vi "Fetch200HZOffsets.vi"(6 "First Segment":dbl, 7 "Number of Segments":dbl, 8 "error in (no error)":errorcluster, 10 "Source (0: Channel 1)":u16(ring) items=["Channel 1", "Channel 2", "Channel 3", "Channel 4"], 11 "VISA Resource Name in":refnum<visa-resource-name>) -> (0 "error out":errorcluster, 2 "HZ offsets":dbl[](array[numeric]), 3 "VISA Resource Name out":refnum<visa-resource-name>)   [LabVIEW 2022 SP3]
uses:
  <instrlib>/LeCroy Wave Series/LeCroy Wave Series.lvlib
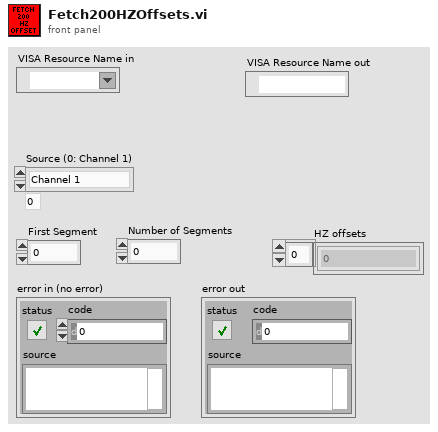
[diagram p1: front panel]
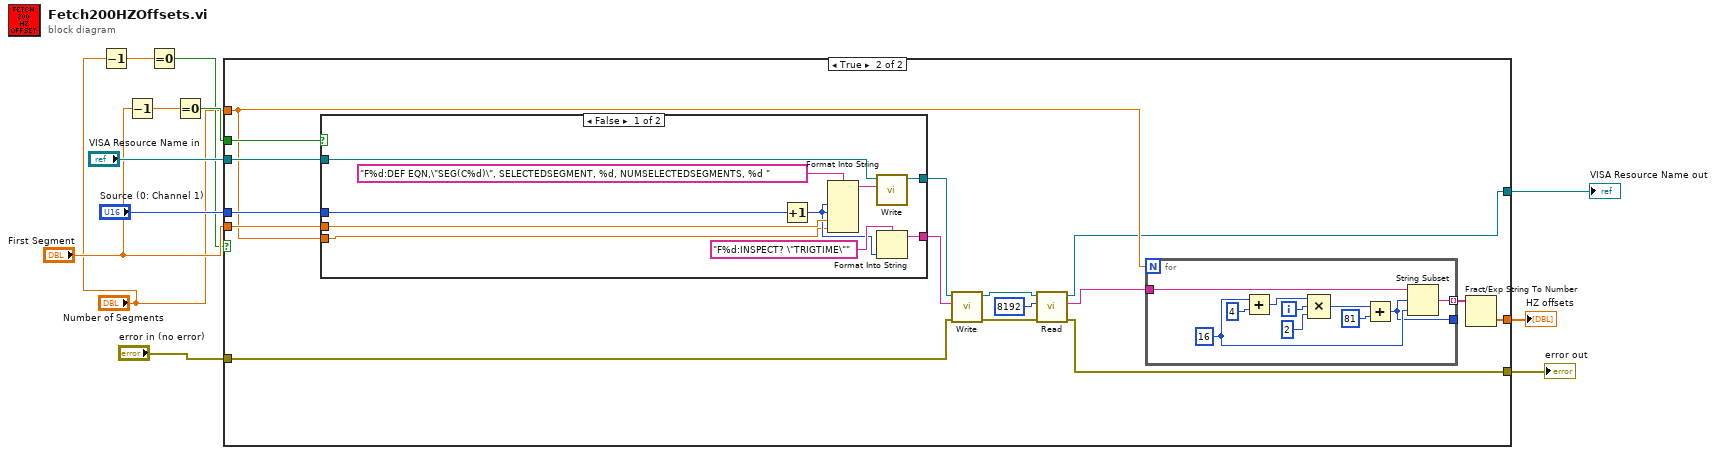
[diagram p0: block diagram]
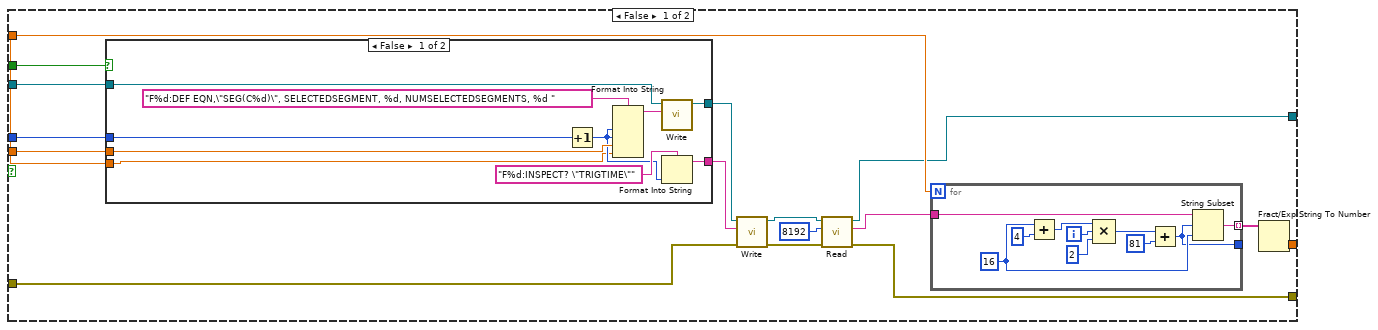
[diagram p2: hidden frame]
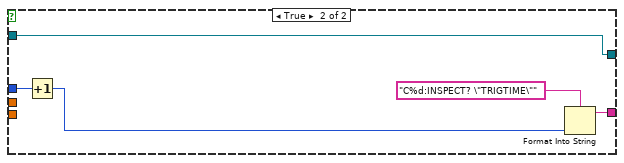
[diagram p3: hidden frame]
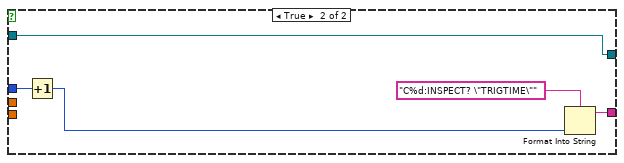
[diagram p4: hidden frame]
diagram:
  n1 = Decrement(x="Number of Segments") -> (x-1=w6:dbl)
  n2 = Decrement(x="First Segment") -> (x-1=w7:dbl)
  n3 = Equal To 0?(x=w6) -> (x = 0?=w5:bool)
  n4 = Equal To 0?(x=w7) -> (x = 0?=w9:bool)
  n5 = case shown="True" w5 {
    tunnel: "Number of Segments" -> [w28 w55]
    tunnel: "VISA Resource Name in" -> [w27 w69]
    tunnel: [w24 w66] -> w11
    tunnel: "Source (0: Channel 1)" -> [w18 w60]
    tunnel: w9 -> [w17 w59]
    tunnel: "First Segment" -> [w16 w58]
    tunnel: "error in (no error)" -> [w15 w56]
    tunnel: [w14 w57] -> w2
    tunnel: [w13 w54] -> w1
    frame False {
      n6 = case shown="False" w17 {
        tunnel: [w37 w43] -> w25
        tunnel: w27 -> [w38 w43]
        tunnel: [w35 w39] -> w26
        tunnel: w16 -> [w33 _]
        tunnel: w28 -> [w30 _]
        tunnel: w18 -> [w34 w40]
        frame False {
          n7 = Increment(x=w34) -> (x+1=w31:u16)
          n8 = Format Into String(format string="F%d:DEF EQN,\"SEG(C%d)\", SELECTEDSEGMENT, %d, NUMSELECTEDSEGMENTS, %d " ("Write Buffer"), w31, w31, w33, w30) -> (resulting string=w32:string)  [unwired: 2 in, 1 out]
          n9 = call <instrlib>:"Write.vi"("Write Buffer"=w32, "VISA resource name"=w38) -> ("VISA resource name out"=w37:refnum<visa-resource-name>)  [unwired: 7 in, 2 out]
          n10 = Format Into String(format string="F%d:INSPECT? \"TRIGTIME\"" ("Write Buffer"), w31) -> (resulting string=w35:string)  [unwired: 2 in, 1 out]
        }
        frame True {
          n11 = Increment(x=w40) -> (x+1=w42:u16)
          n12 = Format Into String(format string="C%d:INSPECT? \"TRIGTIME\"" ("Write Buffer"), w42) -> (resulting string=w39:string)  [unwired: 2 in, 1 out]
        }
      }
      n13 = call <instrlib>:"Write.vi"("error in (no error)"=w15, "Write Buffer"=w26, "VISA resource name"=w25) -> ("error out"=w19:errorcluster, "VISA resource name out"=w20:refnum<visa-resource-name>)  [unwired: 6 in, 1 out]
      n14 = call <instrlib>:"Read.vi"("error in (no error)"=w19, "Byte Count"=u32 8192, "VISA resource name"=w20) -> ("error out"=w14:errorcluster, "Read Buffer"=w22:string, "VISA resource name out"=w13:refnum<visa-resource-name>)  [unwired: 5 in, 1 out]
      n15 = for {
        N: w28 -> [_]
        tunnel: w22 -> [w52]
        tunnel: [w48] -> w23 mode=indexing
        tunnel: [w47] -> _
        i -> [w46]
        w51 = 16 ("length (rest)")
        n16 = Add(x=w51, y=4) -> (x+y=w45:i32)
        n17 = Compound Arithmetic op=MULTIPLY(w45, w46, 2 ("value")) -> (w50:i32)
        n18 = Add(x=w50, y=81 ("offset (0)")) -> (x+y=w47:i32)
        n19 = String Subset(string=w52, offset (0)=w47, length (rest)=w51) -> (substring=w48:string)
      }
      n20 = Fract/Exp String To Number(string=w23) -> (number=w24:dbl[])  [unwired: 3 in, 1 out]
    }
    frame True {
      n21 = case shown="False" w59 {
        tunnel: [w78 w84] -> w67
        tunnel: w69 -> [w79 w84]
        tunnel: [w76 w80] -> w68
        tunnel: w58 -> [w74 _]
        tunnel: w55 -> [w71 _]
        tunnel: w60 -> [w75 w81]
        frame False {
          n22 = Increment(x=w75) -> (x+1=w72:u16)
          n23 = Format Into String(format string="F%d:DEF EQN,\"SEG(C%d)\", SELECTEDSEGMENT, %d, NUMSELECTEDSEGMENTS, %d " ("Write Buffer"), w72, w72, w74, w71) -> (resulting string=w73:string)  [unwired: 2 in, 1 out]
          n24 = call <instrlib>:"Write.vi"("Write Buffer"=w73, "VISA resource name"=w79) -> ("VISA resource name out"=w78:refnum<visa-resource-name>)  [unwired: 7 in, 2 out]
          n25 = Format Into String(format string="F%d:INSPECT? \"TRIGTIME\"" ("Write Buffer"), w72) -> (resulting string=w76:string)  [unwired: 2 in, 1 out]
        }
        frame True {
          n26 = Increment(x=w81) -> (x+1=w83:u16)
          n27 = Format Into String(format string="C%d:INSPECT? \"TRIGTIME\"" ("Write Buffer"), w83) -> (resulting string=w80:string)  [unwired: 2 in, 1 out]
        }
      }
      n28 = call <instrlib>:"Write.vi"("error in (no error)"=w56, "Write Buffer"=w68, "VISA resource name"=w67) -> ("error out"=w61:errorcluster, "VISA resource name out"=w62:refnum<visa-resource-name>)  [unwired: 6 in, 1 out]
      n29 = call <instrlib>:"Read.vi"("error in (no error)"=w61, "Byte Count"=u32 8192, "VISA resource name"=w62) -> ("error out"=w57:errorcluster, "Read Buffer"=w64:string, "VISA resource name out"=w54:refnum<visa-resource-name>)  [unwired: 5 in, 1 out]
      n30 = for {
        N: w55 -> [_]
        tunnel: w64 -> [w93]
        tunnel: [w89] -> w65 mode=indexing
        tunnel: [w88] -> _
        i -> [w87]
        w92 = 16 ("length (rest)")
        n31 = Add(x=w92, y=4) -> (x+y=w86:i32)
        n32 = Compound Arithmetic op=MULTIPLY(w86, w87, 2 ("value")) -> (w91:i32)
        n33 = Add(x=w91, y=81 ("offset (0)")) -> (x+y=w88:i32)
        n34 = String Subset(string=w93, offset (0)=w88, length (rest)=w92) -> (substring=w89:string)
      }
      n35 = Fract/Exp String To Number(string=w65) -> (number=w66:dbl[])  [unwired: 3 in, 1 out]
    }
  }
  "HZ offsets" <- w11
  "error out" <- w2
  "VISA Resource Name out" <- w1
